vi "basci vi_window smoothing.vi"(4 "points to average":i32, 6 "Y":dbl[](array[numeric]), 7 "X":dbl[](array[numeric])) -> (2 "Y smoothed":dbl[](array[numeric]), 3 "X smoothed":dbl[](array[numeric]))   [LabVIEW 2020, in "BasicVIs.lvlib"]
uses:
  BasicVIs.lvlib
  <vilib>/Analysis/baseanly.llb/Mean (DBL).vi
  <vilib>/Analysis/NI_AALBase.lvlib
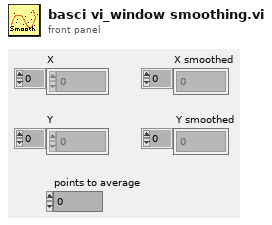
[diagram p1: front panel]
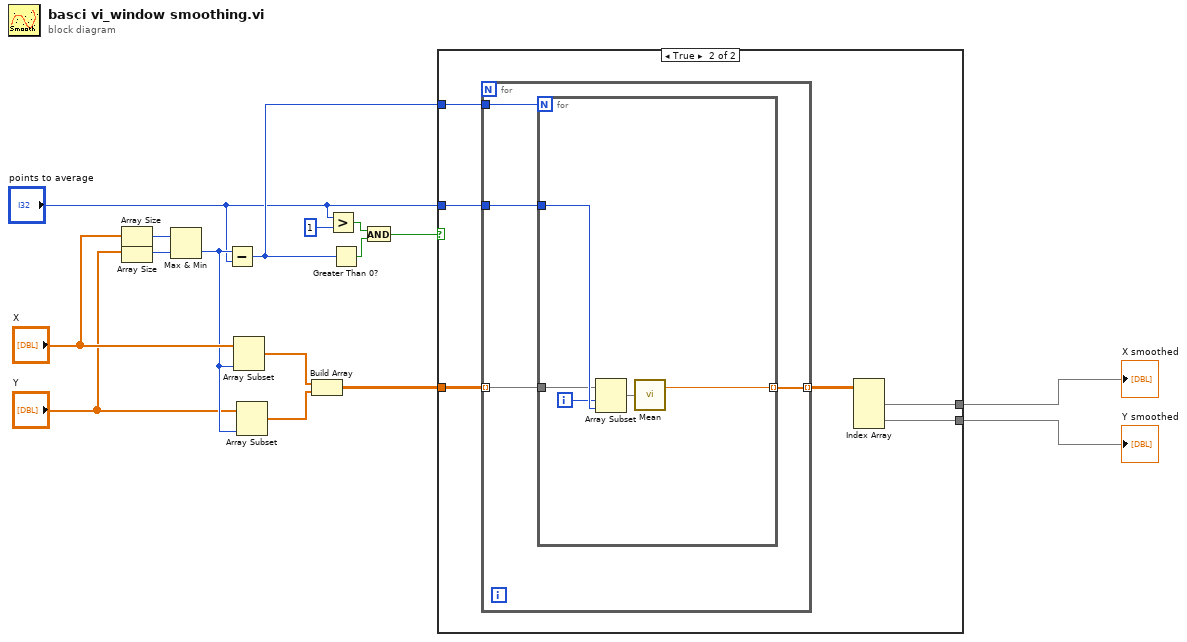
[diagram p0: block diagram]
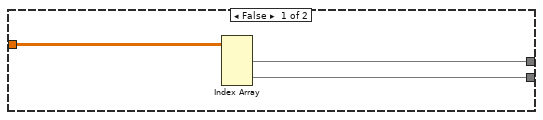
[diagram p2: hidden frame]
diagram:
  n1 = Array Size(array="X") -> (size(s)=w16:i32)
  n2 = Array Size(array="Y") -> (size(s)=w15:i32)
  n3 = Max & Min(x=w16, y=w15) -> (min(x,y)=w12:i32)  [unwired: 1 out]
  n4 = Subtract(x=w12, y="points to average") -> (x-y=w14:i32)
  n5 = Array Subset(array="X", length=w12) -> (w9:dbl[])  [unwired: 1 in]
  n6 = Array Subset(array="Y", length=w12) -> (w10:dbl[])  [unwired: 1 in]
  n7 = Build Array(w9, w10) -> (w8:dbl[][])
  n8 = Greater?(x="points to average", y=1) -> (0:w2:bool)
  n9 = Greater Than 0?(x=w14) -> (x > 0?=w3:bool)
  n10 = And(x=w2, y=w3) -> (x .and. y?=w1:bool)
  n11 = case shown="True" w1 {
    tunnel: w14 -> [_ w25]
    tunnel: w8 -> [w19 w24]
    tunnel: "points to average" -> [_ w23]
    tunnel: [w18 w21] -> w7
    tunnel: [w17 w20] -> w6
    frame False {
      n12 = Index Array(array=w19) -> (element #1=w18:dbl[], element #2=w17:dbl[])  [unwired: 4 in]
    }
    frame True {
      n13 = for {
        tunnel: w25 -> [w29]
        tunnel: w24 -> [w27] mode=indexing
        tunnel: w23 -> [w28]
        tunnel: [w26] -> w22 mode=indexing
        n14 = for {
          N: w29 -> [_]
          tunnel: w28 -> [w34]
          tunnel: w27 -> [w32]
          tunnel: [w30] -> w26 mode=indexing
          i -> [w33]
          n15 = Array Subset(array=w32, index=w33, length=w34) -> (w31:dbl[])
          n16 = call-poly <vilib>:"Mean.vi"("X"=w31) -> ("mean"=w30:dbl)  [unwired: 1 out]
        }
      }
      n17 = Index Array(array=w22) -> (element #1=w21:dbl[], element #2=w20:dbl[])  [unwired: 4 in]
    }
  }
  "X smoothed" <- w7
  "Y smoothed" <- w6
